vi "Save to File Single Channel.vi"(8 "error in (no error)":errorcluster, 11 "File Control":T1) -> (0 "error out":errorcluster)   [LabVIEW 2017]
uses:
  Controls/File Controls.ctl
  <vilib>/Waveform/WDTFileIO.llb/Read Waveform from File.vi
  <vilib>/Utility/file.llb/Write Delimited Spreadsheet (DBL).vi
panel:
  out "Dev1 + Trigger Signals":dbl[][](array[numeric])
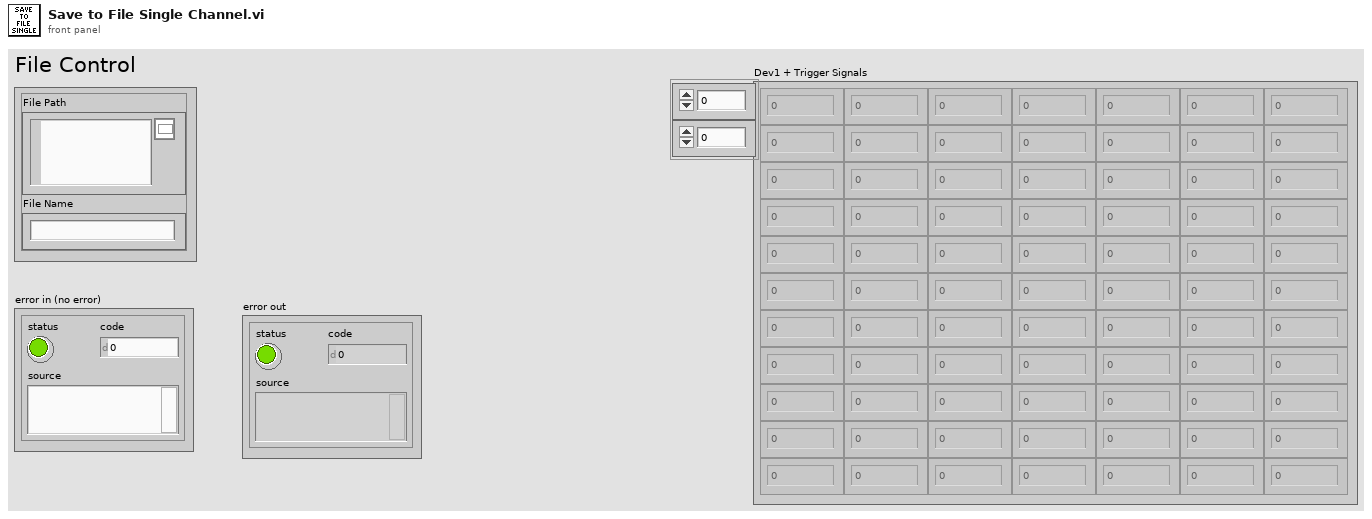
[diagram p1: front panel]
types:
  T1 = typedef "File Controls.ctl" = cluster{"File Path":path, "File Name":string}
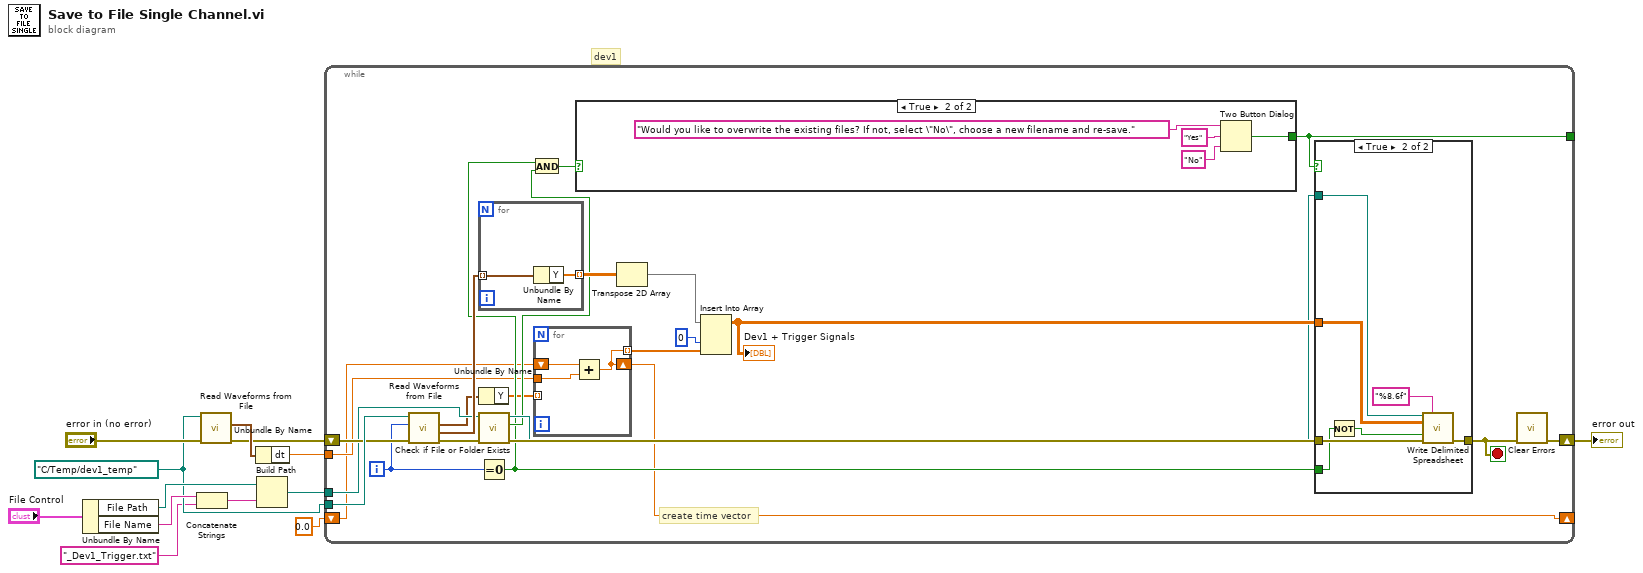
[diagram p0: block diagram]
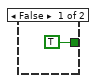
[diagram p2: hidden frame]
diagram:
  w7 = path "C:/Temp/dev1_temp" ("file path (dialog if empty)")
  # "dev1"
  n1 = Unbundle By Name("File Control") -> ("File Path"=w12:path, "File Name"=w11:string)
  n2 = Concatenate Strings(w11, "_Dev1_Trigger.txt" ("string")) -> (w10:string)
  n3 = call-poly <vilib>:"Read Waveforms from File.vi"("error in (no error)"="error in (no error)", "file path (dialog if empty)"=w7) -> ("error out"=w4:errorcluster, "first waveform in record"=w6:waveform(dbl))  [unwired: 4 in, 2 out]
  n4 = Unbundle By Name(w6) -> ("dt"=w5:dbl)
  n5 = Build Path(base path=w12, name or relative path=w10) -> (appended path=w2:path)
  n6 = while {
    tunnel: w7 -> [w37]
    shift-right: [w28] -> w1
    shift-left: w4 -> [w36]
    shift-right: [w15] -> _
    shift-left: 0.0 -> [w17]
    tunnel: w5 -> [w18]
    tunnel: [w23] -> _
    tunnel: w2 -> [w21]
    i -> [w25]
    stop <- w27 stop-if-true
    # "create time vector"
    n7 = call-poly <vilib>:"Read Waveforms from File.vi"("error in (no error)"=w36, "offset (records:0)"=w25, "file path (dialog if empty)"=w37) -> ("error out"=w22:errorcluster, "all waveforms in record"=w35:waveform(dbl)[], "first waveform in record"=w20:waveform(dbl))  [unwired: 3 in, 1 out]
    n8 = for {
      tunnel: w35 -> [w55] mode=indexing
      tunnel: [w54] -> w34 mode=indexing
      n9 = Unbundle By Name(w55) -> ("Y"=w54:dbl[])
    }
    n10 = Unbundle By Name(w20) -> ("Y"=w19:dbl[])
    n11 = call <vilib>:"Check if File or Folder Exists.vi"("error in (no error)"=w22, "path"=w21) -> ("error out"=w31:errorcluster, "file or folder exists?"=w29:bool, "dup path"=w30:path)  [unwired: 7 in]
    n12 = Equal To 0?(x=w25) -> (x = 0?=w24:bool)
    n13 = And(x=w24, y=w29) -> (x .and. y?=w26:bool)
    n14 = for {
      tunnel: w19 -> [_] mode=indexing
      tunnel: w18 -> [w40]
      shift-right: [w38] -> w15
      shift-left: w17 -> [w39]
      tunnel: [w38] -> w16 mode=indexing
      n15 = Add(x=w39, y=w40) -> (x+y=w38:dbl)
    }
    n16 = case shown="True" w26 {
      tunnel: [TRUE ("T button?") w45] -> w23
      frame False {
      }
      frame True {
        n17 = Two Button Dialog(message="Would you like to overwrite the existing files? If not, select \"No\", choose a new filename and re-save.", 1:"No" ("F button name (\"Cancel\")"), 2:"Yes" ("T button name (\"OK\")")) -> (T button?=w45:bool)
      }
    }
    n18 = Transpose 2D Array(2D array=w34) -> (transposed array=w14:dbl[][])
    n19 = Insert Into Array(array=w14, index (col)=0 ("disabled index (col)"), new element=w16) -> (w32:dbl[][])  [unwired: 1 in]
    "Dev1 + Trigger Signals" <- w32
    n20 = case shown="True" w23 {
      tunnel: [w46 w47] -> w27
      tunnel: w32 -> [_ w53]
      tunnel: w30 -> [_ w52]
      tunnel: w31 -> [w46 w51]
      tunnel: w24 -> [_ w49]
      frame False {
      }
      frame True {
        n21 = Not(x=w49) -> (.not. x?=w48:bool)
        n22 = call-poly <vilib>:"Write Delimited Spreadsheet.vi"("file path (dialog if empty)"=w52, "format (%.3f)"="%8.6f", "2D data"=w53, "append to file? (new file:F)"=w48, "error in (no error)"=w51) -> ("error out"=w47:errorcluster)  [unwired: 9 in, 1 out]
      }
    }
    n23 = call <vilib>:"Clear Errors.vi"("error in (no error)"=w27) -> ("error out"=w28:errorcluster)  [unwired: 5 in, 1 out]
  }
  "error out" <- w1
